vi "do MW chop camera frame trigger pulse sequence.vi"(10 "camera frame time (s)":dbl=0.0065, 11 "MW settling time (s)":dbl=0.00152) -> (2 "camera frame time out (s)":dbl=0.0065, 3 "MW settling time out (s)":dbl=0.00152)   [LabVIEW 2019]
panel:
  in  "frame trig ch #":i32=1
  in  "MW ch #":i32=2
  in  "frameburst trig ch #":i32
  in  "Flags (default)":bool[](array[boolean])=[FALSE, FALSE, FALSE, FALSE, FALSE, FALSE, FALSE, FALSE, FALSE, FALSE, FALSE, FALSE, FALSE, FALSE, FALSE, FALSE, FALSE, FALSE, FALSE, FALSE, FALSE, FALSE, FALSE, FALSE]
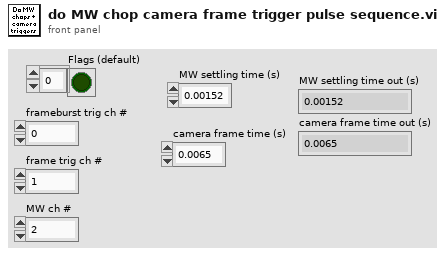
[diagram p1: front panel]
types:
  T1 = enum16{"Pulse Program", "Frequency Registers", "TX Phase Registers", "RX Phase Registers"}
  T2 = cluster{"Instruct Data":i32, "Op Code":i32, "Flags":bool[], "Comments":string, "Time (s)":dbl}
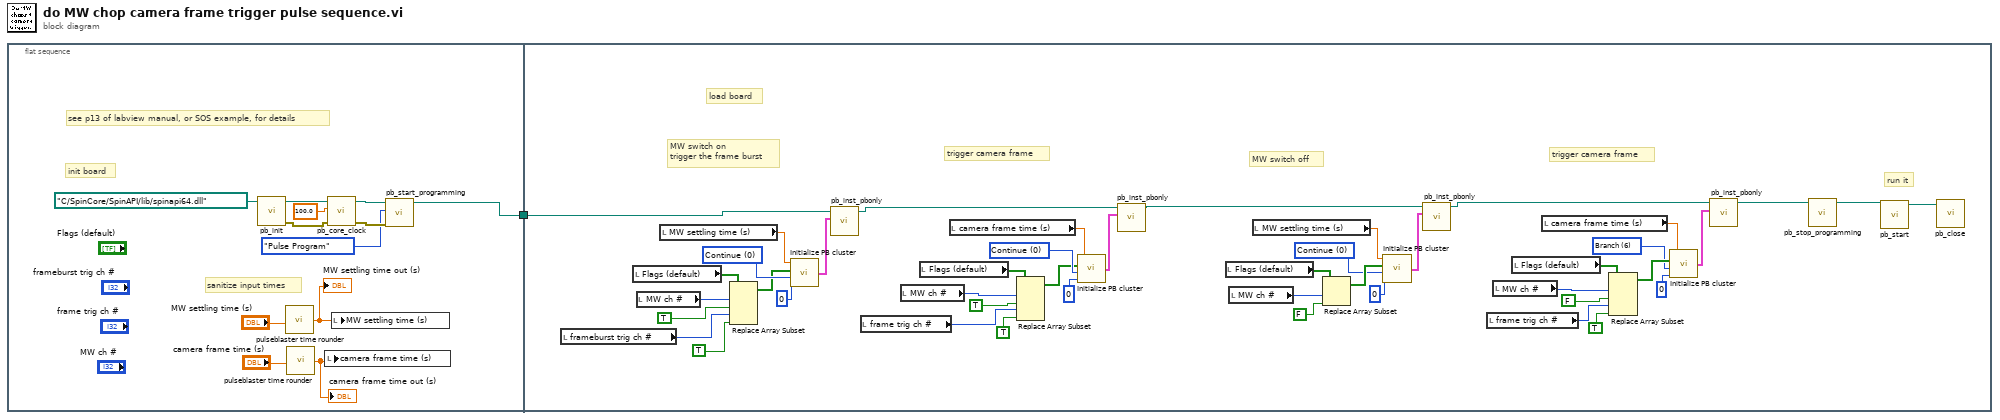
[diagram p0: block diagram]
diagram:
  n1 = flat-sequence {
    tunnel: [w6] -> w1
    tunnel: w1 -> [w58]
    frame #0 {
      # "sanitize input times"
      # "see p13 of labview manual, or SOS example, for details"
      # "init board"
      n2 = call "pb_init.vi"("path in"=path "C:/SpinCore/SpinAPI/lib/spinapi64.dll" ("Location of spinapi.dll")) -> ("error out"=w12:errorcluster, "path out"=w10:path)  [unwired: 3 in, 6 out]
      n3 = call "pulseblaster time rounder.vi"("input time (s)"="MW settling time (s)") -> ("rounded time (s)"=w3:dbl)
      "MW settling time out (s)" <- w3
      n4 = call "pulseblaster time rounder.vi"("input time (s)"="camera frame time (s)") -> ("rounded time (s)"=w2:dbl)
      "camera frame time out (s)" <- w2
      n5 = local write "camera frame time (s)"(w2) -> ()
      n6 = call "pb_core_clock.vi"("error in (no error)"=w12, "clock_freq (MHz)"=100.0, "path in"=w10) -> ("error out"=w13:errorcluster, "path out"=w11:path)  [unwired: 7 in]
      n7 = local write "MW settling time (s)"(w3) -> ()
      n8 = call "pb_start_programming.vi"("error in (no error)"=w13, "Device"=T1."Pulse Program", "path in"=w11) -> ("path out"=w6:path)  [unwired: 1 in, 7 out]
    }
    frame #1 {
      w30 = 0 items=["Continue", "Stop", "Loop", "End Loop", "JSR", "RTS", "Branch", "Long Delay", "Wait"] ("Op Code")
      w21 = 6 items=["Continue", "Stop", "Loop", "End Loop", "JSR", "RTS", "Branch", "Long Delay", "Wait"] ("Op Code")
      w45 = 0 items=["Continue", "Stop", "Loop", "End Loop", "JSR", "RTS", "Branch", "Long Delay", "Wait"] ("Op Code")
      w54 = 0 items=["Continue", "Stop", "Loop", "End Loop", "JSR", "RTS", "Branch", "Long Delay", "Wait"] ("Op Code")
      # "trigger camera frame"
      # "MW switch off"
      # "trigger camera frame"
      # "MW switch on\ntrigger the frame burst"
      # "run it"
      # "load board"
      n9 = local read "frameburst trig ch #"() -> (w14:i32)
      n10 = local read "Flags (default)"() -> (w41:bool[])
      n11 = local read "MW ch #"() -> (w39:i32)
      n12 = local read "MW settling time (s)"() -> (w40:dbl)
      n13 = Replace Array Subset(array=w41, new element #1=TRUE ("new element/subarray"), index #1=w39, new element #2=TRUE ("new element/subarray"), index #2=w14) -> (w43:bool[])
      n14 = call "Initialize PB cluster.vi"("Instruct Data"=0, "Op Code"=w45, "Flags"=w43, "Time (s)"=w40) -> ("PB Instruction"=w46:T2)
      n15 = call "pb_inst_pbonly.vi"("PB Instruction"=w46, "path in"=w58) -> ("path out"=w38:path)  [unwired: 3 in, 6 out]
      n16 = local read "frame trig ch #"() -> (w55:i32)
      n17 = local read "MW ch #"() -> (w51:i32)
      n18 = local read "Flags (default)"() -> (w49:bool[])
      n19 = local read "camera frame time (s)"() -> (w50:dbl)
      n20 = Replace Array Subset(array=w49, new element #1=TRUE ("new element/subarray"), index #1=w51, new element #2=TRUE ("new element/subarray"), index #2=w55) -> (w48:bool[])
      n21 = call "Initialize PB cluster.vi"("Instruct Data"=0, "Op Code"=w54, "Flags"=w48, "Time (s)"=w50) -> ("PB Instruction"=w47:T2)
      n22 = call "pb_inst_pbonly.vi"("PB Instruction"=w47, "path in"=w38) -> ("path out"=w17:path)  [unwired: 3 in, 6 out]
      n23 = local read "Flags (default)"() -> (w34:bool[])
      n24 = local read "MW ch #"() -> (w36:i32)
      n25 = local read "MW settling time (s)"() -> (w35:dbl)
      n26 = Replace Array Subset(array=w34, new element=FALSE ("new element/subarray"), index=w36) -> (w32:bool[])
      n27 = call "Initialize PB cluster.vi"("Instruct Data"=0, "Op Code"=w30, "Flags"=w32, "Time (s)"=w35) -> ("PB Instruction"=w29:T2)
      n28 = call "pb_inst_pbonly.vi"("PB Instruction"=w29, "path in"=w17) -> ("path out"=w37:path)  [unwired: 3 in, 6 out]
      n29 = local read "frame trig ch #"() -> (w20:i32)
      n30 = local read "MW ch #"() -> (w24:i32)
      n31 = local read "Flags (default)"() -> (w26:bool[])
      n32 = local read "camera frame time (s)"() -> (w25:dbl)
      n33 = Replace Array Subset(array=w26, new element #1=FALSE ("new element/subarray"), index #1=w24, new element #2=TRUE ("new element/subarray"), index #2=w20) -> (w27:bool[])
      n34 = call "Initialize PB cluster.vi"("Instruct Data"=0, "Op Code"=w21, "Flags"=w27, "Time (s)"=w25) -> ("PB Instruction"=w28:T2)
      n35 = call "pb_inst_pbonly.vi"("PB Instruction"=w28, "path in"=w37) -> ("path out"=w18:path)  [unwired: 3 in, 6 out]
      n36 = call "pb_stop_programming.vi"("path in"=w18) -> ("path out"=w57:path)  [unwired: 2 in, 8 out]
      n37 = call "pb_start.vi"("path in"=w57) -> ("path out"=w16:path)  [unwired: 2 in, 8 out]
      n38 = call "pb_close.vi"("path in"=w16) -> ()  [unwired: 1 in, 10 out]
    }
  }
